vi "get Data Element.vi"(0 "LVx - Template Command in":refnum<class "REx - NART - Report Calibration Point Power.lvclass">, 11 "error in (no error)":errorcluster) -> (4 "LVx - Template Command out":refnum<class "REx - NART - Report Calibration Point Power.lvclass">, 6 "Power, dB":dbl=62.0, 15 "error out":errorcluster)   [LabVIEW 2011, in "ART2 Test Panel.lvlib" / "REx - NART - Report Calibration Point Power.lvclass"]
uses:
  REx - NART - Calibrate/REx - NART - Report Calibration Point Power.lvclass
  REx - NART - Calibrate/REx - NART - Report Calibration Point Power.lvclass/REx - NART - Report Calibration Point Power.ctl
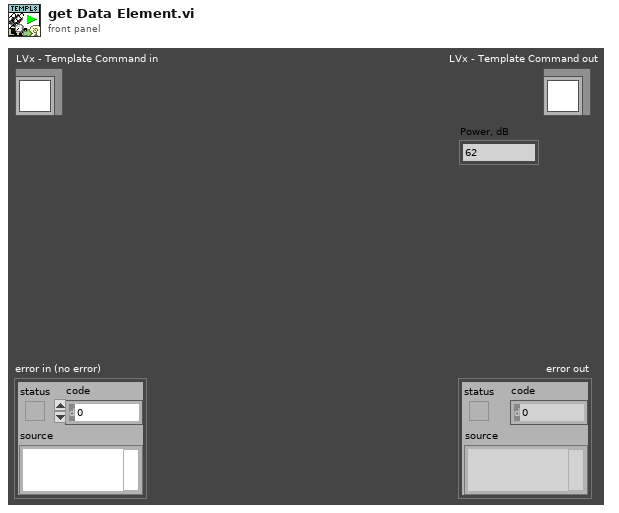
[diagram p1: front panel]
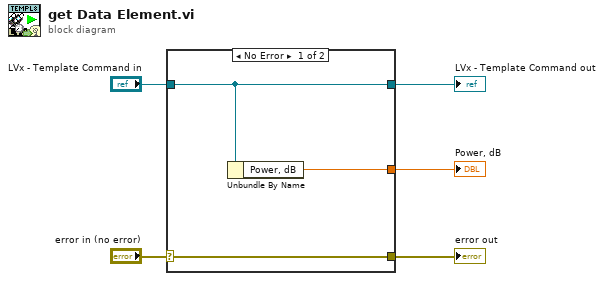
[diagram p0: block diagram]
diagram:
  n1 = case shown="No Error" "error in (no error)" {
    selector: "error in (no error)" -> [w8 w9]
    tunnel: [w8 w9] -> w4
    tunnel: [w6 w10] -> w2
    tunnel: "LVx - Template Command in" -> [w6 w10]
    tunnel: [w7 _] -> w1
    frame No Error {
      n2 = Unbundle By Name(w6) -> ("Power, dB"=w7:dbl)
    }
    frame Error {
    }
  }
  "error out" <- w4
  "LVx - Template Command out" <- w2
  "Power, dB" <- w1
